vi "Display Name.vi"(11 "User BluelinesRedlines in":refnum<class "User BluelinesRedlines.lvclass">) -> (2 "Display Name":string)   [LabVIEW 2020, in "VolatusGUIElements.lvlib" / "User BluelinesRedlines.lvclass"]
uses:
  User BluelinesRedlines.lvclass
  User BluelinesRedlines.lvclass/User BluelinesRedlines.ctl
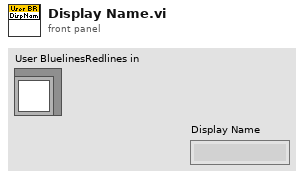
[diagram p1: front panel]
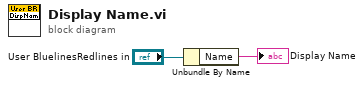
[diagram p0: block diagram]
diagram:
  n1 = Unbundle By Name("User BluelinesRedlines in") -> ("Name"=→"Display Name":string)
